vi "CreatCsv.vi"(8 "error in":errorcluster, 11 "Array":cluster{u16[]}[](array[cluster])) -> (0 "error out":errorcluster)   [LabVIEW 2016]
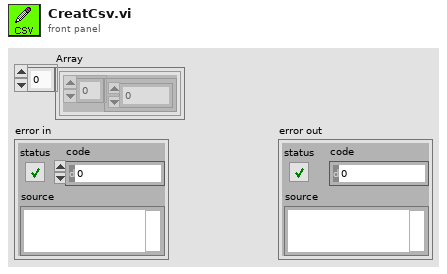
[diagram p1: front panel]
types:
  T1 = enum16{"open", "replace", "create", "open or create", "replace or create", "replace or create with confirmation"}
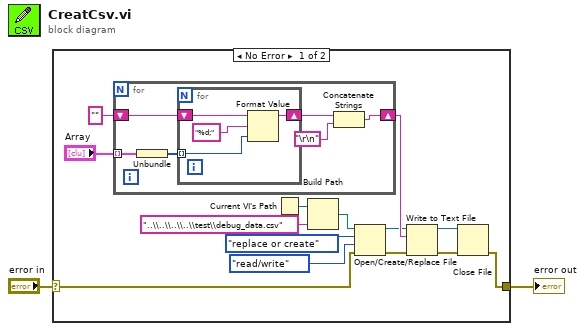
[diagram p0: block diagram]
diagram:
  n1 = case shown="No Error" "error in" {
    selector: "error in" -> [w4 w27]
    tunnel: [w3 w27] -> w1
    frame No Error {
      n2 = for {
        tunnel: "Array" -> [w21] mode=indexing
        shift-right: [w17] -> w14
        shift-left: "" ("string") -> [w22]
        n3 = Unbundle(w21) -> (w20:u16[])
        n4 = for {
          tunnel: w20 -> [w26] mode=indexing
          shift-right: [w23] -> w19
          shift-left: w22 -> [w24]
          n5 = Format Value(string ("")=w24, format string="%d;", value (0)=w26) -> (output string=w23:string)
        }
        n6 = Concatenate Strings(w19, "\r\n") -> (w17:string)
      }
      n7 = Current VI's Path() -> (path=w5:path)
      n8 = Build Path(base path=w5, name or relative path="..\\..\\..\\..\\test\\debug_data.csv") -> (appended path=w9:path)
      n9 = Open/Create/Replace File(file path (use dialog)=w9, error in=w4, operation (0:open)=T1."replace or create", access (0:read/write)=enum16{"read/write", "read-only", "write-only"}."read/write") -> (refnum out=w12:refnum<file>, error out=w13:errorcluster)  [unwired: 2 in, 1 out]
      n10 = Write to Text File(file (use dialog)=w12, text=w14, error in=w13) -> (refnum out=w15:refnum<file>, error out=w16:errorcluster)  [unwired: 1 in, 1 out]
      n11 = Close File(refnum=w15, error in=w16) -> (error out=w3:errorcluster)  [unwired: 1 out]
    }
    frame Error {
    }
  }
  "error out" <- w1
